vi "Passive Force Clamp-final-v2.vi"(4 "file name add to the end (height)":string="h300", 5 "feedback?":bool, 6 "X=T,Y=F":bool=TRUE, 7 "save?":bool, 8 "Set Force (pN)":dbl=45.0 format="%_8g", 9 "moving step size (um)":dbl=0.03, 10 "Auto Find":bool=TRUE, 11 "range (um)":dbl=2.0 format="%.3f") -> ()   [LabVIEW 2014]
uses:
  <vilib>/Analysis/baseanly.llb/Mean (DBL).vi
  <vilib>/Analysis/NI_AALBase.lvlib
panel:
  in  "Tab Control 2":enum32{"Force", "Power"}(tab)
  in  "Intensity Control, 0~-7000 (mV)":dbl=-600.0 format="%_8g"
  out "Lower Pos (um)":dbl
  out "Upper Pos (um)":dbl
  in  "jump (nm)":dbl=195.0
  out "Jump to middle (um)":dbl
  out "Max QPD-Stage Pos (um)":dbl
  in  "lower set value":dbl=0.26
  out "target QPD (V)":dbl
  in  "Avg. time delay (ms)":dbl=20.0
  out "True Target position":dbl
  out "Record scan rate  (um/s)":dbl=2.0
  out "Laser Lock?":bool
  out "Center QPD yc (V)":dbl format="%0.2f"
  out "Sampling rate after filtering (Hz)":dbl
  in  "Who's Data":enum16{"YCC", "PYW", "LCH", "YYH"}(ring)
  out "Stage-QPD data":dbl[][](array[numeric])
  out "Now position (um)":dbl
  in  "Avg points":i32=320
  out "Real initial position (um)":dbl format="%0.5f"
  out "Axis":i32
  in  "toward+ ?\nT=+, F=-":bool
  out "target position (um)":dbl
  in  "upper set value":dbl=0.34
  in  "stop":bool
  in  "Tab Control":T1(tab)
  out "XY Graph":T2(graph)
  in  "Set Target position?":bool
  in  "Custom choose?":bool
  out "Z-QPD":dbl(graph)
  out "Waveform Chart":dbl[](graph)
  out "XY Graph 2":T3(graph)
  out "XY Graph 3":T3(graph)
  in  "Sampling rate":dbl=32000.0
  # "pFC region: jump 170 to 220"
  # "20R-- 300mV"
  # "peak~350 nm\nfrom r = 400 to 500 nm"
  # "jump to r=450 nm"
  # "2.9um for had acted"
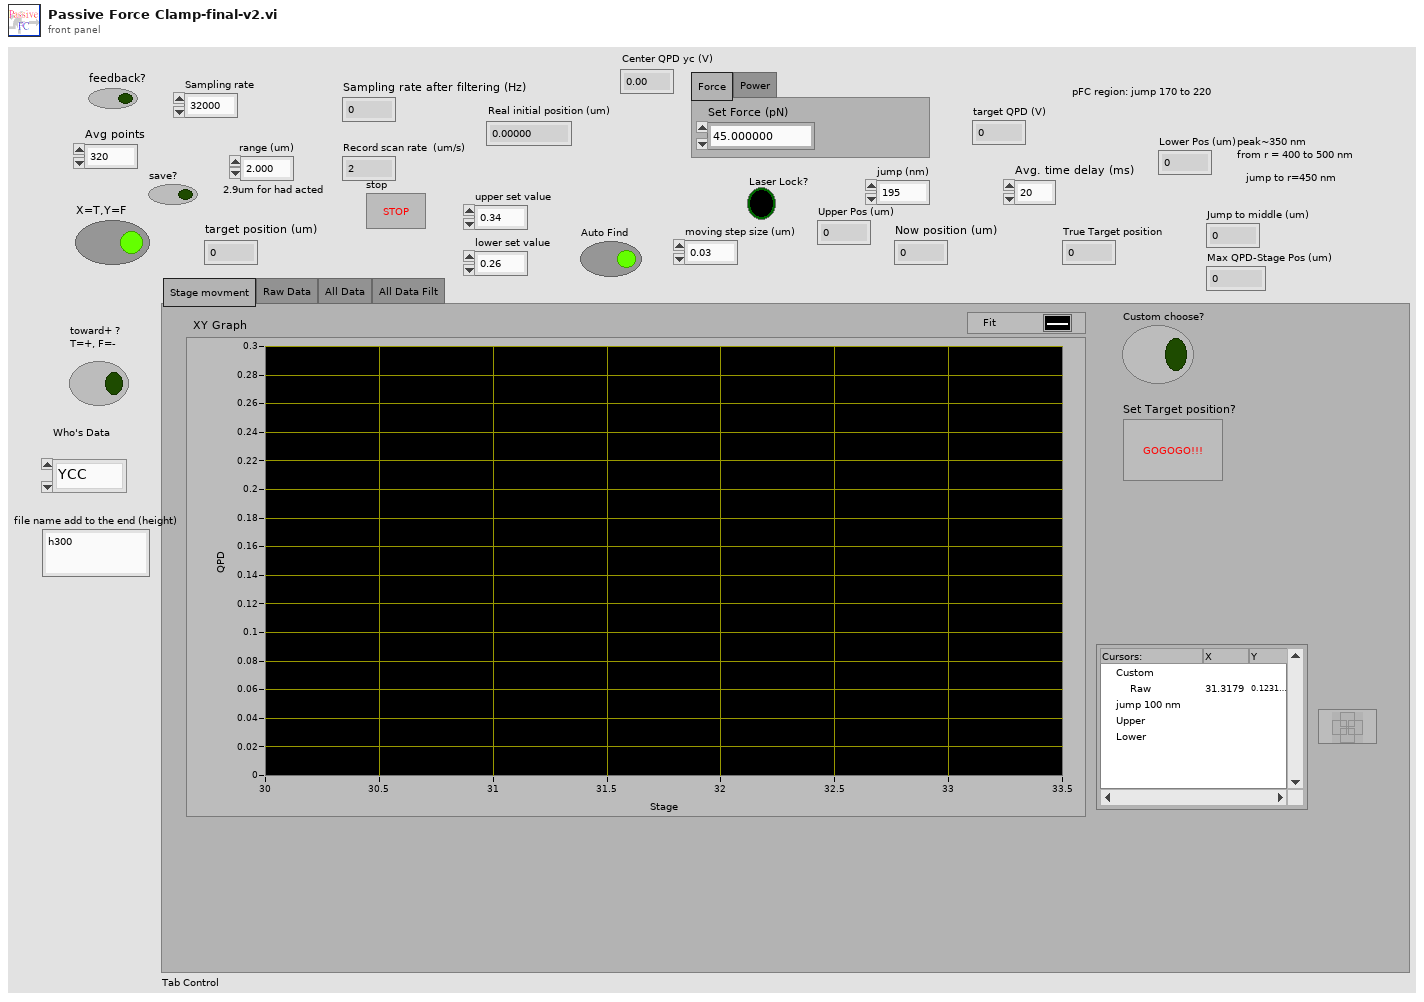
[diagram p1: front panel]
types:
  T1 = enum32{"Stage movment", "Raw Data", "All Data", "All Data Filt"}
  T2 = cluster{"Correct Unfolded Stage Array (um)":dbl[], "Filtered QPD Array":dbl[]}[]
  T3 = cluster{"Time Array (s)":dbl[], "Filtered QPD data":dbl[]}
  T4 = enum16{"Fixed-window avg", "Moving-window avg", "F+S-window avg", "S-G filter", "Fixed-window Median", "Moving-window Median "}
  T5 = cluster{"Correct Unfolded Stage Array (um)":dbl[], "Filtered QPD Array":dbl[]}
  T6 = cluster{"Time Array (s)":dbl[], "Filtered X":dbl[]}
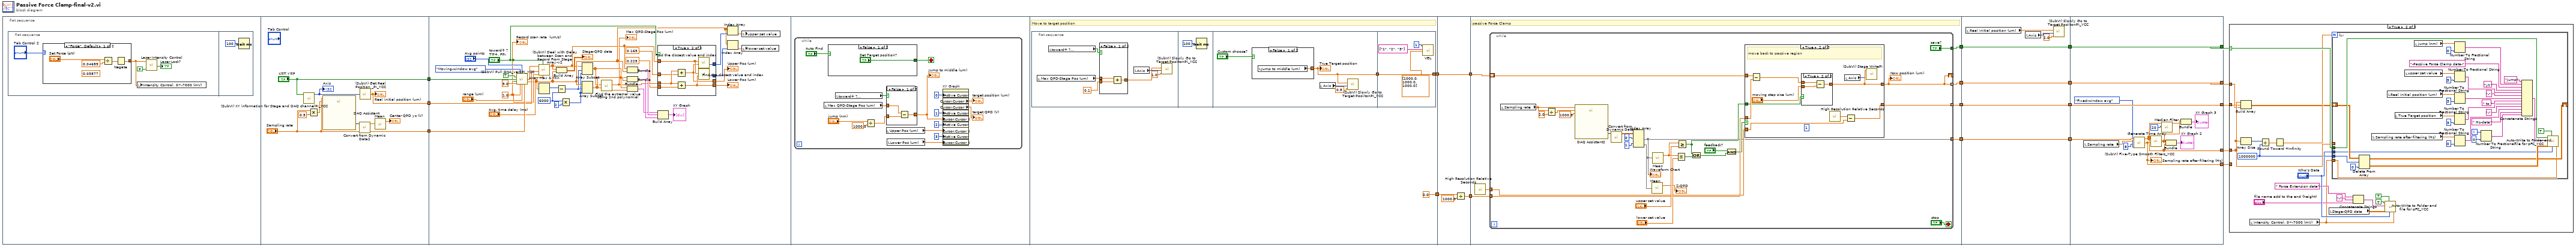
[diagram p0: block diagram]
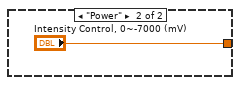
[diagram p3: hidden frame]
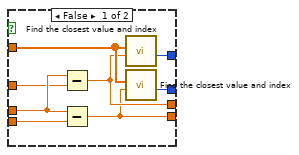
[diagram p4: hidden frame]
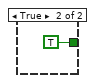
[diagram p5: hidden frame]
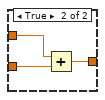
[diagram p6: hidden frame]
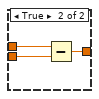
[diagram p7: hidden frame]
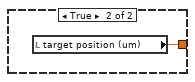
[diagram p8: hidden frame]
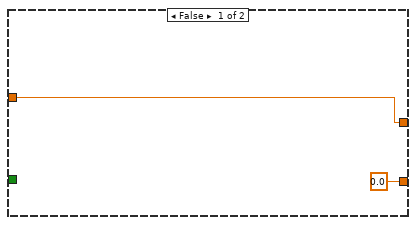
[diagram p9: hidden frame]
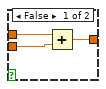
[diagram p10: hidden frame]
diagram:
  n1 = flat-sequence {
    tunnel: [w38] -> w17
    tunnel: ["X=T,Y=F"] -> w16
    tunnel: ["Sampling rate"] -> w5
    tunnel: w17 -> [w67]
    tunnel: w16 -> [w70]
    tunnel: w5 -> [w69]
    tunnel: [w117] -> w15
    tunnel: [0.0 ("Expect - Real move (nm)\nStage Offset\n+=more move\n-=less move")] -> w4
    tunnel: w15 -> [w145]
    tunnel: [w145] -> w14
    tunnel: [w143] -> w13
    tunnel: w4 -> [w142]
    tunnel: w14 -> [w149]
    tunnel: w13 -> [w148]
    tunnel: [w146] -> w11
    tunnel: [w151] -> w9
    tunnel: [w150] -> w7
    tunnel: [w147] -> w2
    tunnel: w11 -> [w203]
    tunnel: [w203] -> w10
    tunnel: w9 -> [w202]
    tunnel: [w202] -> w8
    tunnel: w7 -> [w201]
    tunnel: [w201] -> w6
    tunnel: [w197] -> w3
    tunnel: w2 -> [w197]
    tunnel: [w216] -> w18
    tunnel: [w217] -> w19
    tunnel: [w208] -> w20
    tunnel: w10 -> [w214]
    tunnel: w8 -> [w217]
    tunnel: w6 -> [w216]
    tunnel: [w210] -> w12
    tunnel: w3 -> [w215]
    tunnel: [w215] -> w1
    frame #0 {
      n2 = flat-sequence {
        frame #0 {
          n3 = case shown="\"Force\", Default" "Tab Control 2" {
            tunnel: [w27 "Intensity Control, 0~-7000 (mV)"] -> w21
            frame "Force", Default {
              (unwired) 0.03877 ("y")
              n4 = Divide(x="Set Force (pN)", y=0.04689) -> (x/y=w26:dbl)
              n5 = Negate(x=w26) -> (-x=w27:dbl)
            }
            frame "Power" {
            }
          }
          n6 = local write "Intensity Control, 0~-7000 (mV)"(w21) -> ()
          n7 = call "Laser Intensity Control.vi"("Close?"=FALSE, "Intensity Control, 0~-7000 (mV)"=w21) -> ("Laser Lock?"=→"Laser Lock?":bool)  [unwired: 5 in]
        }
        frame #1 {
          n8 = Wait (ms)(milliseconds to wait=u32 100) -> ()  [unwired: 1 out]
        }
      }
    }
    frame #1 {
      n9 = call "(SubVI) XY information for Stage and DAQ channelPI_YCC.vi"("T=X\nF=Y"="X=T,Y=F") -> ("Axis"=w39:i32)  [unwired: 3 in, 1 out]
      "Axis" <- w39
      n10 = Multiply(x="Sampling rate", y=0.5) -> (x*y=w34:dbl)
      n11 = call "DAQ Assistant"("rate"="Sampling rate", "number of samples"=w34) -> ("data"=w33:dynamicdata)  [unwired: 15 in, 2 out]
      n12 = call "Convert from Dynamic Data2"("Dynamic Data Type"=w33) -> ("Array"=w32:dbl[])  [unwired: 3 in]
      n13 = call "(SubVI) Get Real Position _PI_YCC.vi"("Axis"=w39) -> ("Real Current Commanded position (um)"=w38:dbl)  [unwired: 4 in]
      "Real initial position (um)" <- w38
      n14 = call-poly <vilib>:"Mean.vi"("X"=w32) -> ("mean"=→"Center QPD yc (V)":dbl)  [unwired: 1 out]
    }
    frame #2 {
      w55 = 6000 ("y")
      w66 = 1.0 ("Record scan rate  (um/s)")
      n15 = call "(SubVI) Pull DNA_ver2PI_YCC.vi"("Filter type"=T4."Moving-window avg", "Avg points"="Avg points", "Record?"=TRUE, "T=X\nF=Y"=w70, "Toward  ?\nT=+, F=-"="toward+ ?\nT=+, F=-", "no Record scan rate  (um/s)"=5.0 ("waiting time per point (ms)\nrange from 5ms to 0.167 ms"), "Record scan rate  (um/s)"=w66, "range  (um)"="range (um)", "Sampling rate"=w69) -> ("Filtered Stage Array"=w53:dbl[], "Filtered QPD Array"=w57:dbl[])  [unwired: 4 in, 1 out]
      n16 = call "(SubVI) Deal with Delay between Scan and Record From Stage Array-v2.vi"("Avg. time delay (ms)"="Avg. time delay (ms)", "Toward first ?\nT=+, F=-"="toward+ ?\nT=+, F=-", "Record scan rate  (um/s)"=w66, "Real initial position (um)"=w67, "Unfolded Stage Array (um)"=w53) -> ("Correct Unfolded Stage Array (um)"=w47:dbl[])  [unwired: 2 in, 2 out]
      n17 = Array Max & Min(array=w57) -> (max index (indices)=w56:i32)  [unwired: 3 out]
      n18 = Build Array(w47, w57) -> (→"Stage-QPD data":dbl[][])
      n19 = Subtract(x=w56, y=w55) -> (x-y=w52:i32)
      n20 = Multiply(x=w55, y=2) -> (x*y=w51:i32)
      n21 = Array Subset(array=w47, index=w52, length=w51) -> (w45:dbl[])
      n22 = Array Subset(array=w57, index=w52, length=w51) -> (w46:dbl[])
      n23 = call "Find the extremal value using 2nd polynomial.vi"("Y"=w46, "X"=w45) -> ("Best Polynomial Fit"=w44:dbl[], "Xm"=w42:dbl)  [unwired: 3 in, 1 out]
      "Max QPD-Stage Pos (um)" <- w42
      n24 = Bundle("Correct Unfolded Stage Array (um)"=w47, "Filtered QPD Array"=w57) -> (w50:T5)  [unwired: 1 in]
      n25 = Bundle(w45, w46) -> (w49:cluster{dbl[], dbl[]})  [unwired: 1 in]
      n26 = Bundle(w45, "Best Polynomial Fit"=w44) -> (w43:cluster{dbl[], "Best Polynomial Fit":dbl[]})  [unwired: 1 in]
      n27 = case shown="True" "toward+ ?\nT=+, F=-" {
        tunnel: w42 -> [w83 w91]
        tunnel: w47 -> [w82 w90]
        tunnel: [w81 w89] -> w63
        tunnel: [w80 w88] -> w62
        tunnel: 0.165 ("y") -> [w79 w87]
        tunnel: 0.225 ("y") -> [w78 w86]
        tunnel: [w77 w85] -> w59
        tunnel: [w76 w84] -> w58
        frame False {
          n28 = Subtract(x=w83, y=w79) -> (x-y=w77:dbl)
          n29 = Subtract(x=w83, y=w78) -> (x-y=w76:dbl)
          n30 = call "Find the closest value and index.vi"("Target Value"=w77, "Data"=w82) -> ("Closest Index of Value"=w81:i32)  [unwired: 4 in, 1 out]
          n31 = call "Find the closest value and index.vi"("Target Value"=w76, "Data"=w82) -> ("Closest Index of Value"=w80:i32)  [unwired: 4 in, 1 out]
        }
        frame True {
          n32 = Add(x=w91, y=w87) -> (x+y=w85:dbl)
          n33 = Add(x=w91, y=w86) -> (x+y=w84:dbl)
          n34 = call "Find the closest value and index.vi"("Target Value"=w85, "Data"=w90) -> ("Closest Index of Value"=w89:i32)  [unwired: 4 in, 1 out]
          n35 = call "Find the closest value and index.vi"("Target Value"=w84, "Data"=w90) -> ("Closest Index of Value"=w88:i32)  [unwired: 4 in, 1 out]
        }
      }
      "Upper Pos (um)" <- w59
      "Lower Pos (um)" <- w58
      n36 = Build Array(w43, w50, w49) -> (→"XY Graph":T2)
      n37 = Index Array(array=w57, index=w63) -> (element=w61:dbl)
      n38 = Index Array(array=w57, index=w62) -> (element=w60:dbl)
      n39 = local write "upper set value"(w61) -> ()
      n40 = local write "lower set value"(w60) -> ()
      "Record scan rate  (um/s)" <- w66
    }
    frame #3 {
      n41 = while {
        stop <- w105 stop-if-true
        n42 = local read "Max QPD-Stage Pos (um)"() -> (w102:dbl)
        n43 = case shown="False" "Auto Find" {
          tunnel: ["Set Target position?" TRUE] -> w105
          frame False {
          }
          frame True {
          }
        }
        n44 = local read "toward+ ?\nT=+, F=-"() -> (w100:bool)
        n45 = Divide(x="jump (nm)", y=1000.0) -> (x/y=w97:dbl)
        n46 = case shown="False" w100 {
          tunnel: w102 -> [w112 w115]
          tunnel: w97 -> [w111 w114]
          tunnel: [w110 w113] -> w101
          frame False {
            n47 = Subtract(x=w112, y=w111) -> (x-y=w110:dbl)
          }
          frame True {
            n48 = Add(x=w115, y=w114) -> (x+y=w113:dbl)
          }
        }
        "Jump to middle (um)" <- w101
        n49 = local read "Upper Pos (um)"() -> (w94:dbl)
        n50 = local read "Lower Pos (um)"() -> (w93:dbl)
        n51 = property on="XY Graph" class="XYGraph (strict)"("Active Cursor"=u32 0, "Active Cursor"=u32 1, "Cursor.Cursor X"=w101, "Active Cursor"=u32 2, "Cursor.Cursor X"=w94, "Active Cursor"=u32 3, "Cursor.Cursor X"=w93) -> ("Cursor.Cursor X"=→"target position (um)":dbl, "Cursor.Cursor Y"=→"target QPD (V)":dbl)  [unwired: 2 in, 2 out]
      }
    }
    frame #4 {
      # "Move to target position"
      n52 = flat-sequence {
        tunnel: [w132] -> w116
        tunnel: [w141] -> w117
        tunnel: w116 -> [w141]
        frame #0 {
          n53 = local read "Max QPD-Stage Pos (um)"() -> (w121:dbl)
          n54 = local read "toward+ ?\nT=+, F=-"() -> (w122:bool)
          n55 = case shown="False" w122 {
            tunnel: w121 -> [w127 w130]
            tunnel: [w126 w129] -> w120
            tunnel: 0.1 ("scan rate  (um/s)") -> [w125 w128]
            frame False {
              n56 = Add(x=w127, y=w125) -> (x+y=w126:dbl)
            }
            frame True {
              n57 = Subtract(x=w130, y=w128) -> (x-y=w129:dbl)
            }
          }
          n58 = local read "Axis"() -> (w124:i32)
          n59 = call "(SubVI) Slowly Go to Target PosiitonPI_YCC.vi"("scan rate  (um/s)"=1.0, "axis"=w124, "Target position (um)"=w120) -> ()  [unwired: 4 in, 1 out]
        }
        frame #1 {
          n60 = Wait (ms)(milliseconds to wait=u32 100) -> ()  [unwired: 1 out]
        }
        frame #2 {
          n61 = case shown="False" "Custom choose?" {
            tunnel: [w136 w137] -> w132
            frame False {
              n62 = local read "Jump to middle (um)"() -> (w136:dbl)
            }
            frame True {
              n63 = local read "target position (um)"() -> (w137:dbl)
            }
          }
          "True Target position" <- w132
          n64 = local read "Axis"() -> (w135:i32)
          n65 = call "(SubVI) Slowly Go to Target PosiitonPI_YCC.vi"("scan rate  (um/s)"=0.5, "axis"=w135, "Target position (um)"=w132) -> ()  [unwired: 4 in, 1 out]
        }
        frame #3 {
          n66 = call "VEL.vi"("System no."=1, "Axes to set"=string[] ["1", "2", "3"], "Velocity values"=dbl[] [1000.0, 1000.0, 1000.0]) -> ()  [unwired: 15 in, 2 out]
        }
      }
    }
    frame #5 {
      n67 = Divide(x=w142, y=1000.0) -> (x/y=w143:dbl)
    }
    frame #6 {
      # "passive Force Clamp"
      n68 = call <vilib>:"High Resolution Relative Seconds.vi"() -> ("relative seconds"=w152:dbl)
      n69 = while {
        tunnel: w152 -> [w175]
        tunnel: [w174] -> w151 mode=indexing
        tunnel: [w161] -> w146 mode=concatenating
        tunnel: ["save?"] -> w150
        shift-right: [w153] -> _
        shift-left: w149 -> [w165]
        tunnel: w148 -> [w166]
        tunnel: [w153] -> w147 mode=indexing
        stop <- "stop" stop-if-true
        n70 = local read "Sampling rate"() -> (w169:dbl)
        n71 = Divide(x=w169, y=2.0) -> (x/y=w167:dbl)
        n72 = call "DAQ Assistant2"("rate"=w169, "number of samples"=w167, "timeout (s)"=1000.0) -> ("data"=w172:dynamicdata)  [unwired: 13 in, 3 out]
        n73 = call "Convert from Dynamic Data"("Dynamic Data Type"=w172) -> ("Array"=w164:dbl[][])  [unwired: 3 in]
        n74 = Index Array(array=w164, index (row) #1=0 ("index (row)"), index (row) #2=1 ("index (row)")) -> (element #1=w161:dbl[], element #2=w160:dbl[])  [unwired: 2 in]
        "Waveform Chart" <- w161
        n75 = call-poly <vilib>:"Mean.vi"("X"=w160) -> ("mean"=→"Z-QPD":dbl)  [unwired: 1 out]
        n76 = call-poly <vilib>:"Mean.vi"("X"=w161) -> ("mean"=w177:dbl)  [unwired: 1 out]
        n77 = Less Or Equal?(x=w177, y="lower set value") -> (x <= y?=w156:bool)
        n78 = Greater Or Equal?(x=w177, y="upper set value") -> (x >= y?=w154:bool)
        n79 = Or(x=w154, y=w156) -> (x .or. y?=w155:bool)
        n80 = And(x="feedback?", y=w155) -> (x .and. y?=w157:bool)
        n81 = case shown="True" w157 {
          tunnel: w175 -> [_ w189]
          tunnel: [0.0 w187] -> w174
          tunnel: [w179 w186] -> w153
          tunnel: w166 -> [_ w184]
          tunnel: w165 -> [w179 w182]
          tunnel: w154 -> [_ w181]
          frame False {
          }
          frame True {
            (unwired) 1 ("read #")
            # "move back to passive region"
            n82 = Subtract(x=w182, y=w184) -> (x-y=w183:dbl)
            n83 = case shown="True" w181 {
              tunnel: "moving step size (um)" -> [w191 w196]
              tunnel: [w193 w195] -> w186
              tunnel: w183 -> [w192 w194]
              frame False {
                n84 = Add(x=w192, y=w191) -> (x+y=w193:dbl)
              }
              frame True {
                n85 = Subtract(x=w194, y=w196) -> (x-y=w195:dbl)
              }
            }
            n86 = call <vilib>:"High Resolution Relative Seconds.vi"() -> ("relative seconds"=w188:dbl)
            n87 = local read "Axis"() -> (w185:i32)
            n88 = Subtract(x=w188, y=w189) -> (x-y=w187:dbl)
            n89 = call "(SubVI) Stage WritePI.vi"("axis"=w185, "position"=w186) -> ()  [unwired: 4 in]
          }
        }
        "Now position (um)" <- w153
      }
    }
    frame #7 {
      n90 = local read "Real initial position (um)"() -> (w199:dbl)
      n91 = local read "Axis"() -> (w200:i32)
      n92 = call "(SubVI) Slowly Go to Target PosiitonPI_YCC.vi"("scan rate  (um/s)"=2.0, "axis"=w200, "Target position (um)"=w199) -> ()  [unwired: 4 in, 1 out]
    }
    frame #8 {
      n93 = local read "Sampling rate"() -> (w212:dbl)
      n94 = call "(SubVI) Five-Type Smooth Filters_YCC.vi"("Filter type"=T4."Fixed-window avg", "Avg points"=8, "Sampling rate (Hz)"=w212, "QPD data"=w214) -> ("Sampling rate after filtering (Hz)"=w210:dbl, "Filtered QPD data"=w208:dbl[])  [unwired: 1 in]
      "Sampling rate after filtering (Hz)" <- w210
      n95 = call "Generate Time Array.vi"("Data rate (Hz)"=w210, "Data"=w208) -> ("Time Array (s)"=w207:dbl[])  [unwired: 4 in]
      n96 = call <vilib>:"Median Filter.vi"("left rank"=20, "X"=w208) -> ("Filtered X"=w206:dbl[])  [unwired: 8 in, 1 out]
      n97 = Bundle("Time Array (s)"=w207, "Filtered QPD data"=w208) -> (→"XY Graph 2":T3)  [unwired: 1 in]
      n98 = Bundle("Time Array (s)"=w207, "Filtered X"=w206) -> (→"XY Graph 3":T6)  [unwired: 1 in]
    }
  }
  n99 = case shown="True" w18 {
    selector: w18 -> [_ w235]
    tunnel: w20 -> [_ w231]
    tunnel: w19 -> [_ w230]
    tunnel: w12 -> [_ _]
    tunnel: w1 -> [_ w218]
    frame False {
    }
    frame True {
      w228 = 1000000 ("y")
      n100 = Build Array(w231, w230, w218) -> (w229:dbl[][])
      n101 = Array Size(array=w231) -> (size(s)=w232:i32)
      n102 = local read "Intensity Control, 0~-7000 (mV)"() -> (w219:dbl)
      n103 = Divide(x=w232, y=w228) -> (x/y=w234:dbl)
      n104 = Round Toward +Infinity(x=w234) -> (ceil(x): smallest int >= x=w233:dbl)
      n105 = local read "Stage-QPD data"() -> (w227:dbl[][])
      n106 = for {
        N: w233 -> [_]
        tunnel: w231 -> [_]
        tunnel: w235 -> [w261]
        shift-right: [w247] -> _
        shift-left: w229 -> [w252]
        tunnel: w228 -> [w251]
        tunnel: "Who's Data" -> [w246]
        tunnel: w219 -> [w241]
        i -> [w259]
        n107 = Delete From Array(array=w252, length=w251, index (col)=0 ("index (row)")) -> (deleted portion=w249:dbl[][], array with subset deleted=w247:dbl[][])  [unwired: 1 in]
        n108 = local read "Sampling rate after filtering (Hz)"() -> (w260:dbl)
        n109 = local read "Real initial position (um)"() -> (w270:dbl)
        n110 = local read "True Target position"() -> (w267:dbl)
        n111 = local read "upper set value"() -> (w244:dbl)
        n112 = local read "jump (nm)"() -> (w239:dbl)
        n113 = Number To Fractional String(number=w239, precision (6)=i16 0) -> (F-format string=w236:string)  [unwired: 2 in]
        n114 = Number To Fractional String(number=w244, precision (6)=i16 5) -> (F-format string=w242:string)  [unwired: 2 in]
        n115 = Number To Fractional String(number=w270, precision (6)=i16 3) -> (F-format string=w266:string)  [unwired: 2 in]
        n116 = Number To Fractional String(number=w267, precision (6)=i16 3) -> (F-format string=w264:string)  [unwired: 2 in]
        n117 = Number To Fractional String(number=w260, precision (6)=i16 0) -> (F-format string=w255:string)  [unwired: 2 in]
        n118 = Number To Fractional String(number=w259, precision (6)=i16 0) -> (F-format string=w253:string)  [unwired: 2 in]
        n119 = Concatenate Strings("jump" ("string"), w236, "-Passive Force Clamp data-" ("prompt"), "yt " ("string"), w242, "-" ("string"), w266, " to " ("string"), w264, "-" ("string"), w255, " Hz-data" ("string"), w253) -> (w262:string)
        n120 = call "Auto-Write to Folder and file for pFC_YCC.vi"("Current PD (mV)"=w241, "Who's Data"=w246, "T=2D\nF=1D"=TRUE ("T=2D\nF=1D"), "2D data to be saved"=w249, "File name add to the end \n(height)"=w262, "Save?"=w261) -> ()  [unwired: 2 in, 2 out]
      }
      n121 = Concatenate Strings(" Force Extension data" ("prompt"), "-" ("string"), "file name add to the end (height)") -> (w220:string)
      n122 = call "Auto-Write to Folder and file for pFC_YCC.vi"("Current PD (mV)"=w219, "Who's Data"="Who's Data", "T=2D\nF=1D"=TRUE ("T=2D\nF=1D"), "2D data to be saved"=w227, "File name add to the end \n(height)"=w220, "Save?"=TRUE) -> ()  [unwired: 2 in, 2 out]
    }
  }
